vi "Resolve Service.vi"(8 "error in":errorcluster, 11 "request data":T1) -> (0 "error out":errorcluster, 3 "response data":T2)   [LabVIEW 2020, in "MeasurementLink Discovery Client Wrapper.lvlib"]
uses:
  MeasurementLink Discovery Client Wrapper.lvlib
  Action.ctl
  MeasurementLink Discovery Client/MeasurementLink Discovery Client.lvlib
  MeasurementLink Discovery Client/RPC Messages/ni_measurementlink_discovery_v1_ServiceLocation.ctl
  MeasurementLink Discovery Client/RPC Messages/ni_measurementlink_discovery_v1_ResolveServiceRequest.ctl
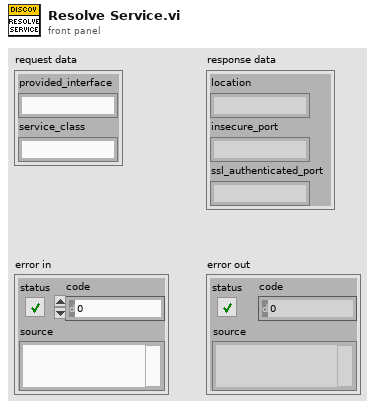
[diagram p1: front panel]
types:
  T1 = typedef "MeasurementLink Discovery Client.lvlib/ni_measurementlink_discovery_v1_ResolveServiceRequest.ctl" = cluster{"provided_interface":string, "service_class":string}
  T2 = typedef "MeasurementLink Discovery Client.lvlib/ni_measurementlink_discovery_v1_ServiceLocation.ctl" = cluster{"location":string, "insecure_port":string, "ssl_authenticated_port":string}
  T3 = typedef "MeasurementLink Discovery Client Wrapper.lvlib/Action.ctl" = enum16{"Get Client", "Destroy Client"}
  T4 = typedef "grpc-lvsupport-release.lvlib/grpcId.ctl" = u64
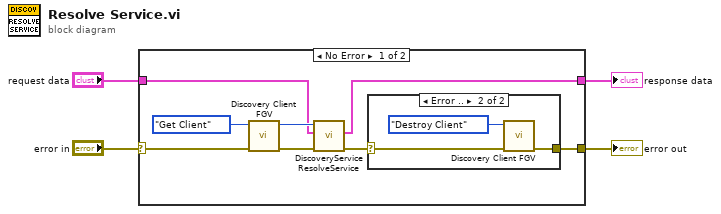
[diagram p0: block diagram]
diagram:
  n1 = case shown="No Error" "error in" {
    selector: "error in" -> [w12 w17]
    tunnel: [w5 w17] -> w3
    tunnel: [w8 _] -> w2
    tunnel: "request data" -> [w7 _]
    frame No Error {
      n2 = call "Discovery Client FGV.vi"("error in"=w12, "action"=Action."Get Client") -> ("error out"=w10:errorcluster, "grpc client id"=w9:T4)  [unwired: 8 in]
      n3 = call "DiscoveryService ResolveService.vi"("error in"=w10, "Request Data"=w7, "gRPC ID"=w9) -> ("error out"=w6:errorcluster, "Response Data"=w8:T2)  [unwired: 6 in, 1 out]
      n4 = case shown="Error .." w6 {
        selector: w6 -> [w13 w16]
        tunnel: [w13 w15] -> w5
        frame No Error {
        }
        frame Error {
          n5 = call "Discovery Client FGV.vi"("error in"=w16, "action"=Action."Destroy Client") -> ("error out"=w15:errorcluster)  [unwired: 8 in, 1 out]
        }
      }
    }
    frame Error {
    }
  }
  "error out" <- w3
  "response data" <- w2
